vi "RegloPumpenDriver.vi"(6 "VISA resource name In":refnum<visa-resource-name>="COM1", 7 "Expected terminator":string="[*+-\\r]", 8 "error in":errorcluster, 10 "Befehl":string caption="Commands (without CR)", 11 "Pump":T1) -> (0 "error out":errorcluster, 1 "Antwort":string caption="Answer without terminator", 2 "Sendstring":string, 3 "Receivestring":string, 4 "VISA resource name Out":refnum<visa-resource-name>)   [LabVIEW 2021]
doc: "Low-Level-Treiber fürdas Messgerät Nivel 20 von Leica Geosystems.\nBenutzt die Default-Baudrate von 9600 Baud.\n\n6. Februar 2003 / av"
uses:
  Pumpen.ctl
  <vilib>/Instr/_visa.llb/VISA Configure Serial Port (Instr).vi
panel:
  in  "Demo-Mode?":bool
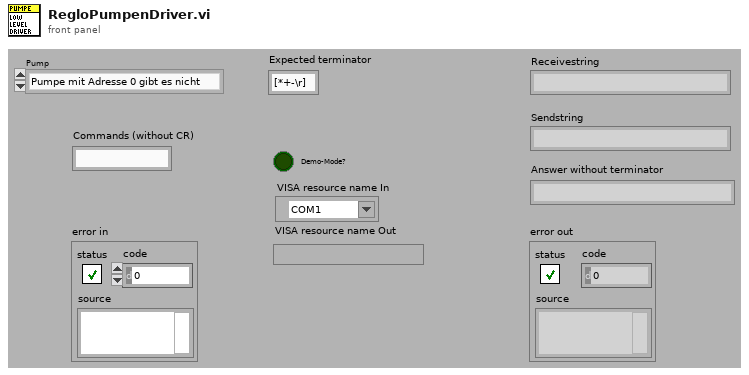
[diagram p1: front panel]
types:
  T1 = typedef "Pumpen.ctl" = enum16{"Pumpe mit Adresse 0 gibt es nicht", "P_01", "P_02", "P_03", "P_04", "P_05", "P_06", "P_07", "P_08"}
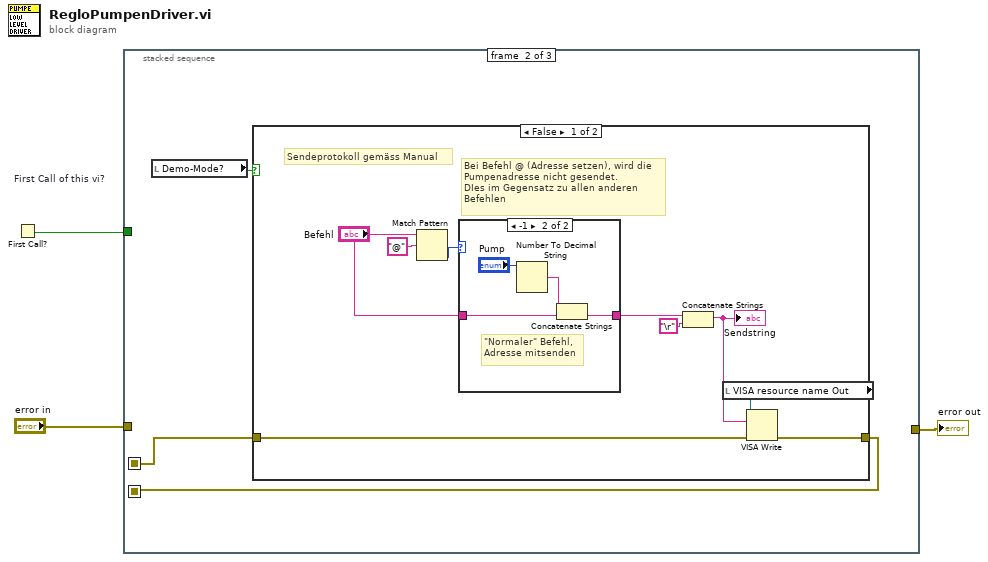
[diagram p0: block diagram]
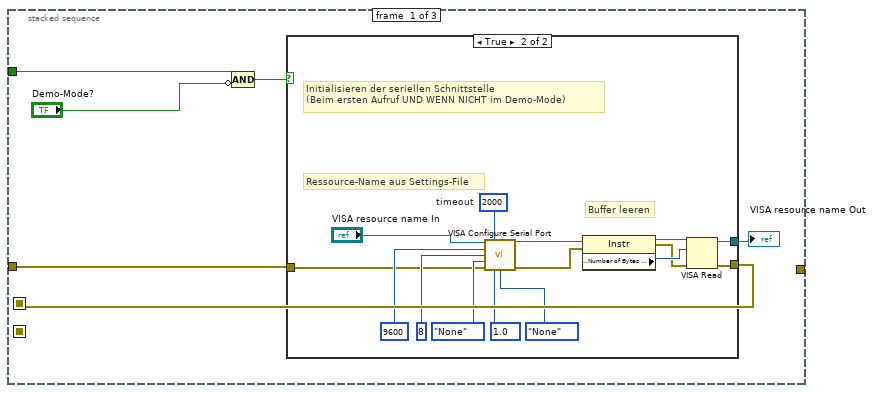
[diagram p2: hidden frame]
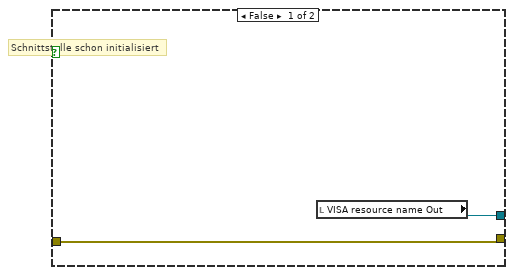
[diagram p3: hidden frame]
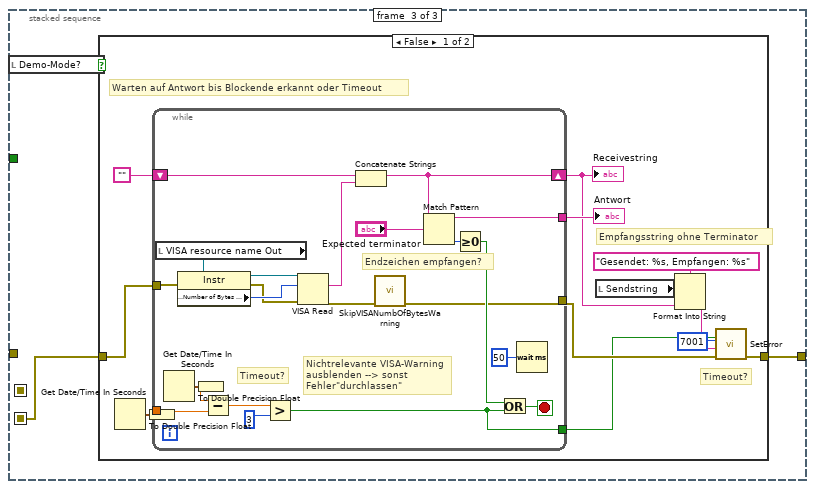
[diagram p6: hidden frame]
diagram:
  n1 = First Call? "First Call of this vi?"() -> (First Call?: T/F=w1:bool)
  n2 = stacked-sequence {
    seq-local: [w9 _ _] -> [_ w29 _]
    seq-local: [_ w28 _] -> [_ _ w47]
    tunnel: "error in" -> [w7 _ _]
    tunnel: [_ _ w46] -> w2
    tunnel: w1 -> [w6 _ _]
    frame #0 {
      n3 = Compound Arithmetic op=AND(w6, invert "Demo-Mode?") -> (w5:bool)
      n4 = case shown="True" w5 {
        tunnel: w7 -> [w11 w13]
        tunnel: [w11 w15] -> w9
        tunnel: [w10 w14] -> w8
        frame False {
          # "Schnittstelle schon initialisiert"
          n5 = local read "VISA resource name Out"() -> (w10:refnum<visa-resource-name>)
        }
        frame True {
          w24 = u16 10 items=["1.0"=10, "1.5"=15, "2.0"=20] ("stop bits (10: 1 bit)")
          w22 = u32 2000  # timeout
          # "Ressource-Name aus Settings-File"
          # "Buffer leeren"
          # "Initialisieren der seriellen Schnittstelle\n(Beim ersten Aufruf UND WENN NICHT im Demo-Mode)"
          n6 = call-poly "VISA Configure Serial Port"("VISA resource name"="VISA resource name In", "timeout (10sec)"=w22, "baud rate (9600)"=u32 9600, "data bits (8)"=u16 8, "parity (0:none)"=enum16{"None", "Odd", "Even", "Mark", "Space"}."None", "error in (no error)"=w13, "stop bits (10: 1 bit)"=w24, "flow control (0:none)"=enum16{"None", "XON/XOFF", "RTS/CTS"}."None" ("flow control (0:None)")) -> ("VISA resource name out"=w17:refnum<visa-resource-name>, "error out"=w16:errorcluster)  [unwired: 6 in]
          n7 = property class="Instr"(reference=w17, error in=w16) -> (reference out=w20:refnum<visa-resource-name>, error out=w18:errorcluster, "Serial Settings:Number of Bytes at Serial Port"=w19:u32)
          n8 = VISA Read(VISA resource name=w20, byte count=w19, error in (no error)=w18) -> (VISA resource name out=w14:refnum<visa-resource-name>, error out=w15:errorcluster)  [unwired: 2 out]
        }
      }
      "VISA resource name Out" <- w8
    }
    frame #1 {
      n9 = local read "Demo-Mode?"() -> (w27:bool)
      n10 = case shown="False" w27 {
        tunnel: w29 -> [w38 w44]
        tunnel: [w36 w44] -> w28
        frame False {
          # "Sendeprotokoll gemäss Manual"
          # "Bei Befehl @ (Adresse setzen), wird die Pumpenadresse nicht gesendet.\nDIes im Gegensatz zu allen anderen Befehlen"
          n11 = Match Pattern(string="Befehl", regular expression="@") -> (offset past match=w33:i32)  [unwired: 1 in, 3 out]
          n12 = case shown="-1" w33 {
            tunnel: [w39 w43] -> w32
            tunnel: "Befehl" -> [w39 w40]
            frame Default {
              # "Bei Befehl enthält \"@\""
            }
            frame -1 {
              # "\"Normaler\" Befehl,\nAdresse mitsenden"
              n13 = Number To Decimal String(number="Pump") -> (decimal integer string=w41:string)  [unwired: 1 in]
              n14 = Concatenate Strings(w41, w40) -> (w43:string)
            }
          }
          n15 = Concatenate Strings(w32, "\r") -> (w34:string)
          "Sendstring" <- w34
          n16 = local read "VISA resource name Out"() -> (w37:refnum<visa-resource-name>)
          n17 = VISA Write(VISA resource name=w37, write buffer=w34, error in (no error)=w38) -> (error out=w36:errorcluster)  [unwired: 2 out]
        }
        frame True {
          # "Demo-Mode"
        }
      }
    }
    frame #2 {
      n18 = local read "Demo-Mode?"() -> (w45:bool)
      n19 = case shown="False" w45 {
        tunnel: w47 -> [w60 w83]
        tunnel: [w57 w83] -> w46
        frame False {
          # "Timeout?"
          # "Empfangsstring ohne Terminator"
          # "Warten auf Antwort bis Blockende erkannt oder Timeout"
          n20 = Get Date/Time In Seconds() -> (seconds since 1Jan1904=w48:timestamp)
          n21 = To Double Precision Float(number=w48) -> (double precision float=w58:dbl)
          n22 = while {
            tunnel: [w67] -> w53
            tunnel: w58 -> [w71]
            shift-left: "" -> [w77]
            shift-right: [w75] -> w51
            tunnel: w60 -> [w80]
            tunnel: [w62] -> w56
            tunnel: [w66] -> w55
            stop <- w72 stop-if-true
            # "Nichtrelevante VISA-Warning\nausblenden --> sonst Fehler\"durchlassen\""
            # "Timeout?"
            # "Endzeichen empfangen?"
            n23 = local read "VISA resource name Out"() -> (w78:refnum<visa-resource-name>)
            n24 = Get Date/Time In Seconds() -> (seconds since 1Jan1904=w61:timestamp)
            n25 = property class="Instr"(reference=w78, error in=w80) -> (reference out=w82:refnum<visa-resource-name>, error out=w64:errorcluster, "Serial Settings:Number of Bytes at Serial Port"=w81:u32)
            n26 = To Double Precision Float(number=w61) -> (double precision float=w70:dbl)
            n27 = Subtract(x=w70, y=w71) -> (x-y=w69:dbl)
            n28 = Greater?(x=w69, y=3) -> (0:w66:bool)
            n29 = VISA Read(VISA resource name=w82, byte count=w81, error in (no error)=w64) -> (read buffer=w76:string, error out=w63:errorcluster)  [unwired: 2 out]
            n30 = Concatenate Strings(w77, w76) -> (w75:string)
            n31 = call "SkipVISANumbOfBytesWarning.vi"("error in (no error)"=w63) -> ("error out"=w62:errorcluster)  [unwired: 9 in, 1 out]
            n32 = Match Pattern(string=w75, regular expression="Expected terminator") -> (before substring=w67:string, offset past match=w74:i32)  [unwired: 1 in, 2 out]
            n33 = Greater Or Equal To 0?(x=w74) -> (x >= 0?=w73:bool)
            n34 = Or(x=w73, y=w66) -> (x .or. y?=w72:bool)
            n35 = Wait (ms)(milliseconds to wait=u32 50) -> ()  [unwired: 1 out]
          }
          "Receivestring" <- w51
          "Antwort" <- w53
          n36 = local read "Sendstring"() -> (w49:string)
          n37 = Format Into String(format string="Gesendet: %s, Empfangen: %s", w49, w51) -> (resulting string=w50:string)  [unwired: 2 in, 1 out]
          n38 = call "SetError.vi"("error in"=w56, "Zusatzinfo zum Fehler"=w50, "error code"=u32 7001, "Error?"=w55) -> ("error out"=w57:errorcluster)  [unwired: 5 in]
        }
        frame True {
          # "Demo-Mode"
        }
      }
    }
  }
  "error out" <- w2
